vi "CS-4 Set Limits.vi"(4 "voltage limit":dbl format="%.2f", 5 "error in (no error)":errorcluster, 6 "lower limit":dbl format="%.2f", 7 "upper limit":dbl format="%.2f", 8 "VISA session":refnum<visa-resource-name>) -> (0 "error out":errorcluster, 3 "dup VISA session":refnum<visa-resource-name>)   [LabVIEW 2016]
doc: "CS-4 Set Limits.vi sets the LOWER and UPPER current limits to be used with the sweep comand."
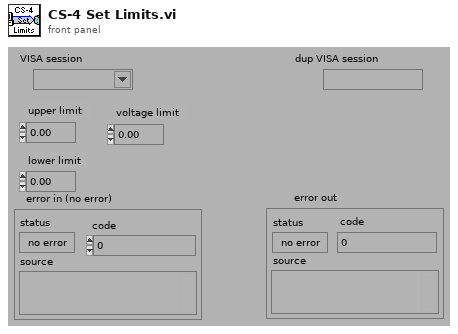
[diagram p1: front panel]
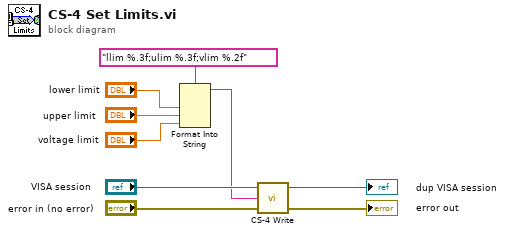
[diagram p0: block diagram]
diagram:
  n1 = Format Into String(format string="llim %.3f;ulim %.3f;vlim %.2f", "lower limit", "upper limit", "voltage limit") -> (resulting string=w1:string)  [unwired: 2 in, 1 out]
  n2 = call "CS-4 Write.vi"("error in (no error)"="error in (no error)", "write buffer (\"\")"=w1, "VISA session"="VISA session") -> ("error out"=→"error out":errorcluster, "dup VISA session"=→"dup VISA session":refnum<visa-resource-name>)  [unwired: 1 out]
